vi "Game_ResetWinnings.vi"(8 "error in (no error)":errorcluster, 11 "Players array":T1[](array[typedef])) -> (0 "error out":errorcluster, 3 "Players array OUT":T1[](array[typedef]))   [LabVIEW 2020]
uses:
  Typedefs/game_player.ctl
  Typedefs/enumeratedPlayers.ctl
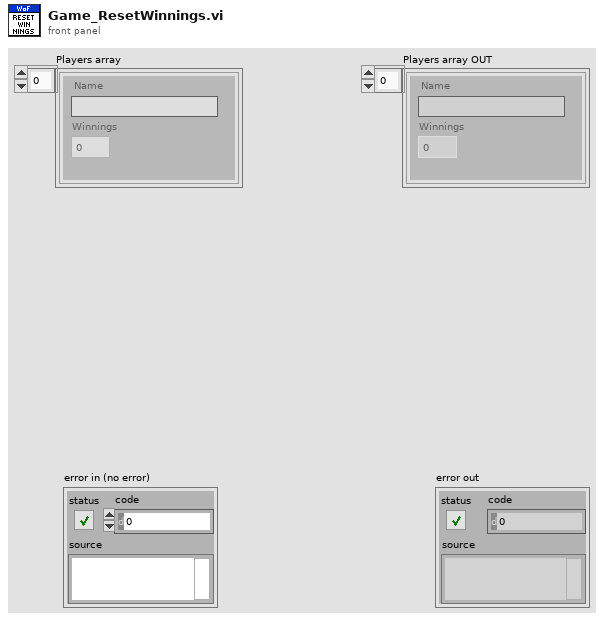
[diagram p1: front panel]
types:
  T1 = typedef "game_player.ctl" = cluster{"Name":string, "Winnings":dbl}
  T2 = typedef "enumeratedPlayers.ctl" = enum16{"one", "two", "three"}
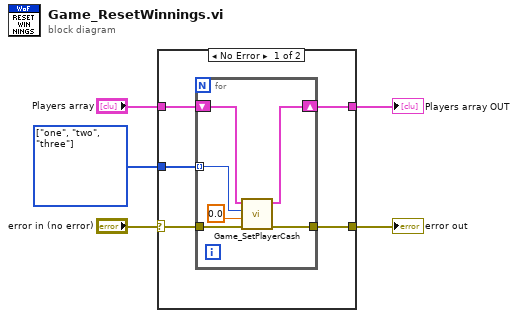
[diagram p0: block diagram]
diagram:
  w4 = T2[] [enum."one", enum."two", enum."three"] items=["one", "two", "three"]
  n1 = case shown="No Error" "error in (no error)" {
    selector: "error in (no error)" -> [w8 w17]
    tunnel: w4 -> [w9 _]
    tunnel: "Players array" -> [w10 w18]
    tunnel: [w7 w17] -> w2
    tunnel: [w6 w18] -> w1
    frame No Error {
      n2 = for {
        shift-right: [w12] -> w6
        shift-left: w10 -> [w13]
        tunnel: w9 -> [w14] mode=indexing
        tunnel: w8 -> [w16]
        tunnel: [w15] -> w7
        n3 = call "Game_SetPlayerCash.vi"("error in (no error)"=w16, "Amount"=0.0, "player"=w14, "Players array"=w13) -> ("error out"=w15:errorcluster, "Players array OUT"=w12:T1[])  [unwired: 6 in]
      }
    }
    frame Error {
    }
  }
  "error out" <- w2
  "Players array OUT" <- w1
